vi "initialise.vi"(8 "error in (no error)":errorcluster, 11 "DAQmxDigitalOut in":refnum<class "DigitalOutDL110325DAQmx.lvclass">) -> (0 "error out":errorcluster, 3 "DAQmxDigitalOut out":refnum<class "DigitalOutDL110325DAQmx.lvclass">)   [LabVIEW 2010, in "DigitalOutDL110325DAQmx.lvclass"]
doc: "The dynamic dispatch-version of this VI initalises the plug-in object by allocating and initalising any dynamic resources need."
uses:
  DigitalOutDL110325DAQmx.lvclass
  GenericDigitalOut/GenericDigitalOut/GenericDigitalOut.lvclass
  DigitalOutDL110325DAQmx.lvclass/DigitalOutDL110325DAQmx.ctl
  <vilib>/DAQmx/create/channels.llb/DAQmx Create Channel (DO-Digital Output).vi
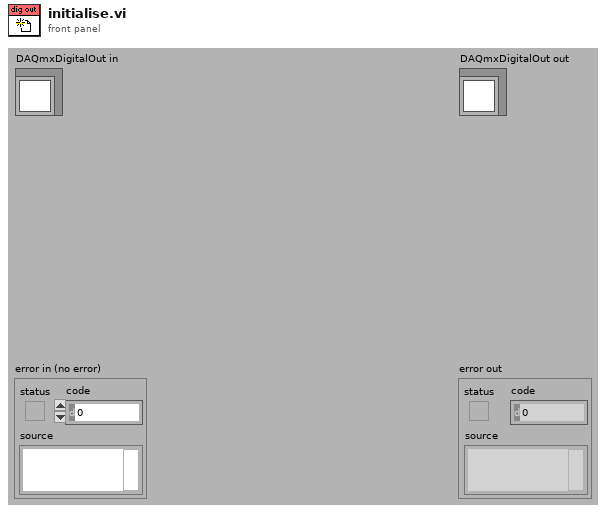
[diagram p1: front panel]
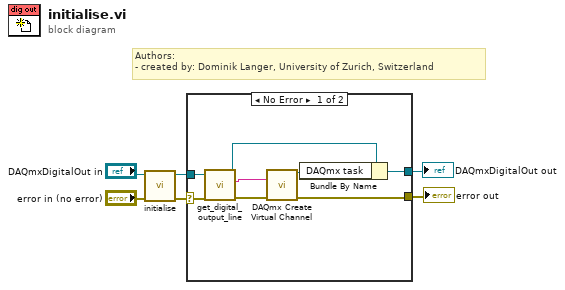
[diagram p0: block diagram]
diagram:
  # "Authors: \n- created by: Dominik Langer, University of Zurich, Switzerland"
  n1 = call-parent "initialise.vi"("error in (no error)"="error in (no error)", "GenericPlugin in"="DAQmxDigitalOut in") -> ("error out"=w4:errorcluster, "GenericPlugin out"=w3:refnum<class "DigitalOutDL110325DAQmx.lvclass">)  [unwired: 8 out]
  n2 = case shown="No Error" w4 {
    selector: w4 -> [w14 w15]
    tunnel: w3 -> [w13 w16]
    tunnel: [w8 w16] -> w2
    tunnel: [w7 w15] -> w1
    frame No Error {
      n3 = call "get_digital_output_line.vi"("error in (no error)"=w14, "DAQmxDigitalOut in"=w13) -> ("error out"=w11:errorcluster, "digital output line"=w12:tag, "DAQmxDigitalOut out"=w9:refnum<class "DigitalOutDL110325DAQmx.lvclass">)  [unwired: 7 out]
      n4 = call-poly <vilib>:"DAQmx Create Virtual Channel.vi"("lines"=w12, "error in"=w11) -> ("task out"=w10:refnum<k21>, "error out"=w7:errorcluster)  [unwired: 3 in, 9 out]
      n5 = Bundle By Name(cluster=w9, "DAQmx task"=w10) -> (w8:refnum<class "DigitalOutDL110325DAQmx.lvclass">)
    }
    frame Error {
    }
  }
  "error out" <- w1
  "DAQmxDigitalOut out" <- w2
